vi "Teleop.vi"(10 "Match Info":T1={"Autonomous Elapsed Seconds"=0.0, "TeleOp Elapsed Seconds"=0.0, "Disabled Elapsed Seconds"=0.0, "Visited Autonomous"=FALSE, "Visited TeleOp"=FALSE, "Visited Disabled"=FALSE, "Autonomous Settings"={"Autonomous Style"=enum."Independent", "VI Refnum"=refnum}}, 11 "Call Context":T2) -> ()   [LabVIEW 2023]
doc: "This VI is called for each TeleOp packet received from the DS where the robot is not disabled. It is often used to read from the joysticks and update I/O or to update setpoints for timed control loops. It should complete and return within 20 milliseconds or it may miss DS packets."
uses:
  <vilib>/Rock Robotics/WPI/DriverStation/WPI_DriverStationDerivedRobotMode.ctl
  <vilib>/Rock Robotics/WPI/DriverStation/WPI_DriverStationMatch Info.ctl
  <vilib>/Rock Robotics/WPI/DriverStation/WPI_DriverStationAllianceInfo.ctl
  1688fe70-1696-4b7d-9b30-3e57ff5c803a.vi
  01ea3398-5322-4b29-8113-0a99e2c097c5.vi
  2d160a00-edc5-41ad-b49c-64d9a7043442.vi
  <vilib>/Rock Robotics/WPI/ThirdParty/JAS_Junk/TrajLib/ProfiledPIDController_NewPeriod.vi
  <vilib>/Rock Robotics/WPI/ThirdParty/JAS_Junk/TrajLib/ProfiledPIDController_SetIntegratorRange.vi
  <vilib>/Rock Robotics/WPI/ThirdParty/JAS_Junk/TrajLib/ProfiledPIDController_DisableContInput.vi
  <vilib>/Rock Robotics/WPI/ThirdParty/JAS_Junk/TrajLib/ProfiledPIDController_EnableContInput.vi
  <vilib>/Rock Robotics/WPI/ThirdParty/JAS_Junk/TrajLib/TrapProfConstraint_New.vi
  <vilib>/Rock Robotics/WPI/ThirdParty/PhotonVisionLib/SubVI/PhotonPipelineResult_Unpack.vi
  <vilib>/Rock Robotics/WPI/ThirdParty/PhotonVisionLib/SubVI/PhotonPipelineResult_SetTimeStampSecs.vi
  <vilib>/Rock Robotics/WPI/ThirdParty/PhotonVisionLib/SubVI/PhotonPipelineResult_GetLatency_Millis.vi
  <vilib>/Rock Robotics/WPI/ThirdParty/JAS_Junk/TrajLib/Util_GetTime.vi
  <vilib>/Rock Robotics/WPI/ThirdParty/PhotonVisionLib/SubVI/PhotonPipelineResult_GetTimeStampSecs.vi
  <vilib>/Rock Robotics/WPI/ThirdParty/JAS_Junk/TrajLib/MathUtil_AngleModulus.vi
  <vilib>/Rock Robotics/WPI/ThirdParty/JAS_Junk/TrajLib/Pose2d_New.vi
  <vilib>/Rock Robotics/WPI/ThirdParty/JAS_Junk/TrajLib/HolDrvCtrl_New.vi
  <vilib>/Rock Robotics/WPI/ThirdParty/JAS_Junk/TrajLib/HolDrvCtrl_PackPID.vi
  <vilib>/Rock Robotics/WPI/ThirdParty/JAS_Junk/TrajLib/HolDrvCtrl_SetTolerance.vi
  <vilib>/Rock Robotics/WPI/ThirdParty/JAS_Junk/TrajLib/HolDrvCtrl_SetEnabled.vi
  <vilib>/Rock Robotics/WPI/ThirdParty/JAS_Junk/TrajLib/HolDrvCtrl_AtReference.vi
  <vilib>/Rock Robotics/WPI/ThirdParty/JAS_Junk/TrajLib/HolDrvCtrl_Calculate.vi
  <vilib>/Rock Robotics/WPI/ThirdParty/JAS_Junk/TrajLib/Rotation2d_RotateBy.vi
  <vilib>/Rock Robotics/WPI/ThirdParty/JAS_Junk/TrajLib/SlewRateLimiter_New.vi
  <vilib>/Rock Robotics/WPI/ThirdParty/JAS_Junk/TrajLib/SlewRateLimiter_Reset.vi
  <vilib>/Rock Robotics/WPI/ThirdParty/JAS_Junk/TrajLib/SlewRateLimiter_Calculate.vi
  <vilib>/Rock Robotics/WPI/ThirdParty/JAS_Junk/TrajLib/SlewRateLimiter_SetRate.vi
  <vilib>/Rock Robotics/WPI/ThirdParty/JAS_Junk/TrajLib/Rotation2d_GetCos.vi
  <vilib>/Rock Robotics/WPI/ThirdParty/JAS_Junk/TrajLib/Rotation2d_GetSin.vi
  <vilib>/Rock Robotics/WPI/ThirdParty/JAS_Junk/TrajLib/ChassisSpeeds_New.vi
  <vilib>/Rock Robotics/WPI/ThirdParty/JAS_Junk/TrajLib/TrapProfState_New.vi
  <vilib>/Rock Robotics/WPI/ThirdParty/JAS_Junk/TrajLib/PIDController_NewPeriod.vi
  <vilib>/Rock Robotics/SystemInterfaces/NetworkCommunication/NetComm_UsageReport_report.vi
  <vilib>/Rock Robotics/WPI/ThirdParty/JAS_Junk/TrajLib/PIDController_SetIntegratorRange.vi
  <vilib>/Rock Robotics/WPI/ThirdParty/JAS_Junk/TrajLib/PIDController_DisableContinousInput.vi
  <vilib>/Rock Robotics/WPI/ThirdParty/JAS_Junk/TrajLib/PIDController_EnableContinousInput.vi
  <vilib>/Rock Robotics/WPI/ThirdParty/PhotonVisionLib/SubVI/Packet_decode_Flt64.vi
  <vilib>/Rock Robotics/WPI/ThirdParty/PhotonVisionLib/SubVI/Packet_decode_ByteI8.vi
  <vilib>/Rock Robotics/WPI/ThirdParty/PhotonVisionLib/SubVI/PhotonTrackedTarget_Unpack.vi
  <vilib>/Rock Robotics/WPI/ThirdParty/PhotonVisionLib/SubVI/PhotonMultiTargetPNPResult_unpack.vi
  <vilib>/Rock Robotics/WPI/ThirdParty/PhotonVisionLib/SubVI/PhotonPipelineResult_New.vi
  <vilib>/Rock Robotics/WPI/ThirdParty/JAS_Junk/TrajLib/VI/Util_GetTime_U32.vi
  <vilib>/Rock Robotics/WPI/ThirdParty/JAS_Junk/TrajLib/MathUtil_InputModulus.vi
  <vilib>/Rock Robotics/WPI/ThirdParty/JAS_Junk/TrajLib/Translation2d_Create.vi
  <vilib>/Rock Robotics/WPI/ThirdParty/JAS_Junk/TrajLib/PIDController_Reset.vi
  <vilib>/Rock Robotics/WPI/ThirdParty/JAS_Junk/TrajLib/Pose2d_getXYAngle.vi
  <vilib>/Rock Robotics/WPI/ThirdParty/JAS_Junk/TrajLib/Rotation2d_GetRadians.vi
  <vilib>/Rock Robotics/WPI/ThirdParty/JAS_Junk/TrajLib/Rotation2d_GetAngleCosSin.vi
  <vilib>/Rock Robotics/WPI/ThirdParty/JAS_Junk/TrajLib/Pose2d_RelativeTo.vi
  <vilib>/Rock Robotics/WPI/ThirdParty/JAS_Junk/TrajLib/Pose2d_getRotation.vi
  <vilib>/Rock Robotics/WPI/ThirdParty/JAS_Junk/TrajLib/Rotation2d_Minus.vi
  <vilib>/Rock Robotics/WPI/ThirdParty/JAS_Junk/TrajLib/ProfiledPIDController_Calculate_Meas_Goal.vi
  <vilib>/Rock Robotics/WPI/ThirdParty/JAS_Junk/TrajLib/PIDController_Calculate_SP_PV.vi
  <vilib>/Rock Robotics/WPI/ThirdParty/JAS_Junk/TrajLib/ProfiledPIDController_Reset_PosOnly.vi
  <vilib>/Rock Robotics/WPI/ThirdParty/JAS_Junk/TrajLib/Rotation2d_CreateXY.vi
  <vilib>/Rock Robotics/WPI/ThirdParty/PhotonVisionLib/SubVI/TargetCorner_New.vi
  <vilib>/Rock Robotics/WPI/ThirdParty/PhotonVisionLib/SubVI/Packet_decode_Int32.vi
  <vilib>/Rock Robotics/WPI/ThirdParty/PhotonVisionLib/SubVI/Packet_decode_Transform3d.vi
  <vilib>/Rock Robotics/WPI/ThirdParty/PhotonVisionLib/SubVI/PhotonPNPResult_unpackt.vi
  <vilib>/Rock Robotics/WPI/ThirdParty/PhotonVisionLib/SubVI/PhotonMultiTargetPNPResult_New.vi
  <vilib>/Rock Robotics/WPI/ThirdParty/PhotonVisionLib/SubVI/PhotonMultiTargetPNPResult_MAX_IDS.vi
  <vilib>/Rock Robotics/WPI/ThirdParty/PhotonVisionLib/SubVI/Packet_decode_Int16.vi
  <vilib>/Rock Robotics/WPI/ThirdParty/JAS_Junk/TrajLib/Transform2d_Create_PosePose.vi
  <vilib>/Rock Robotics/WPI/ThirdParty/JAS_Junk/TrajLib/Pose2d_New_TRRO.vi
  <vilib>/Rock Robotics/WPI/ThirdParty/JAS_Junk/TrajLib/Rotation2d_UnaryMinus.vi
  <vilib>/Rock Robotics/WPI/ThirdParty/JAS_Junk/TrajLib/ProfiledPIDController_SetGoal_PosOnly.vi
  <vilib>/Rock Robotics/WPI/ThirdParty/JAS_Junk/TrajLib/ProfiledPIDController_Calculate_Meas.vi
  <vilib>/Rock Robotics/WPI/ThirdParty/JAS_Junk/TrajLib/PIDController_SetSetpoint.vi
  <vilib>/Rock Robotics/WPI/ThirdParty/JAS_Junk/TrajLib/PIDController_Calculate_PV.vi
  <vilib>/Rock Robotics/WPI/ThirdParty/JAS_Junk/TrajLib/ProfiledPIDController_Reset.vi
  <vilib>/Rock Robotics/WPI/ThirdParty/JAS_Junk/TrajLib/Util_CalcDist.vi
  <vilib>/Rock Robotics/WPI/ThirdParty/JAS_Junk/TrajLib/VI/Transform3d_Create_Trans3dRot3d.vi
  <vilib>/Rock Robotics/WPI/ThirdParty/JAS_Junk/TrajLib/VI/Translation3d_Create.vi
  <vilib>/Rock Robotics/WPI/ThirdParty/JAS_Junk/TrajLib/VI/Rotation3d_Create_Quaternion.vi
  <vilib>/Rock Robotics/WPI/ThirdParty/JAS_Junk/TrajLib/VI/Quaternion_New.vi
  <vilib>/Rock Robotics/WPI/ThirdParty/PhotonVisionLib/SubVI/Packet_decode_Boolean.vi
  <vilib>/Rock Robotics/WPI/ThirdParty/PhotonVisionLib/SubVI/PhotonPNPResult_New_Empty.vi
  <vilib>/Rock Robotics/WPI/ThirdParty/PhotonVisionLib/SubVI/PhotonPNPResult_New.vi
  <vilib>/Rock Robotics/WPI/ThirdParty/JAS_Junk/TrajLib/Translation2d_RotateBy.vi
  <vilib>/Rock Robotics/WPI/ThirdParty/JAS_Junk/TrajLib/Translation2d_Minus.vi
  <vilib>/Rock Robotics/WPI/ThirdParty/JAS_Junk/TrajLib/ProfiledPIDController_SetGoal.vi
  <vilib>/Rock Robotics/WPI/ThirdParty/JAS_Junk/TrajLib/TrapProfile_New.vi
  <vilib>/Rock Robotics/WPI/ThirdParty/JAS_Junk/TrajLib/ProfiledPIDController_GetPeriod.vi
  <vilib>/Rock Robotics/WPI/ThirdParty/JAS_Junk/TrajLib/TrapProfile_Calculate.vi
  <vilib>/Rock Robotics/WPI/ThirdParty/JAS_Junk/TrajLib/ControllerUtil_GetModulusError.vi
  <vilib>/Rock Robotics/WPI/ThirdParty/JAS_Junk/TrajLib/VI/Quaternion_Normalize.vi
  <vilib>/Rock Robotics/WPI/ThirdParty/JAS_Junk/TrajLib/TrapProfile_ShouldFlipAcceleration.vi
  <vilib>/Rock Robotics/WPI/ThirdParty/JAS_Junk/TrajLib/TrapProfile_Direct.vi
  <vilib>/Rock Robotics/WPI/ThirdParty/JAS_Junk/TrajLib/PIDController_GetPeriod.vi
  <vilib>/Rock Robotics/WPI/ThirdParty/JAS_Junk/TrajLib/VI/Quaternion_New_Default.vi
  <vilib>/Rock Robotics/Network Tables/NT Read Boolean.vi
  <vilib>/Rock Robotics/Network Tables/NT Read Number.vi
  <vilib>/Rock Robotics/WPI/Utilities/WPI_GetSetVariantRefNum.vi
  <vilib>/Rock Robotics/Network Tables/NT Write Boolean Array.vi
  <vilib>/Rock Robotics/Network Tables/NT Write Numeric Array.vi
  <vilib>/Rock Robotics/Network Tables/NT Write String.vi
  <vilib>/Rock Robotics/Network Tables/NT Read String.vi
  <vilib>/Rock Robotics/Network Tables/NT Write Boolean.vi
  <vilib>/Rock Robotics/Network Tables/NT Write Number.vi
  <vilib>/Rock Robotics/WPI/ThirdParty/JAS_Junk/TrajLib/Globals/Util_LibraryGlobals.vi
  <vilib>/Rock Robotics/Network Tables/NT Read Raw.vi
  <vilib>/Rock Robotics/WPI/ThirdParty/JAS_Junk/TrajLib/VI/Util_GetTime_U64.vi
  Swerve_Drive_System/SWERVE_DRIVE_GLOBALS.vi
  <vilib>/addons/control/pid/pid.llb/PID Control Input Filter (DBL).vi
  <vilib>/Rock Robotics/WPI/ThirdParty/JAS_Junk/TrajLib/Trajectory_Library.lvlib
  55d04a09-3dfb-4cd7-90e5-cf451b4756f2.vi
  <vilib>/addons/control/pid/NI_PID_pid.lvlib
  <vilib>/Rock Robotics/WPI/ThirdParty/PhotonVisionLib/PhotonVisionLib.lvlib
panel:
  out "Sample Slider 0":dbl(slide) scale=0.0..5.0
  out "Sample Boolean 1":bool
  out "Sample Boolean 0":bool
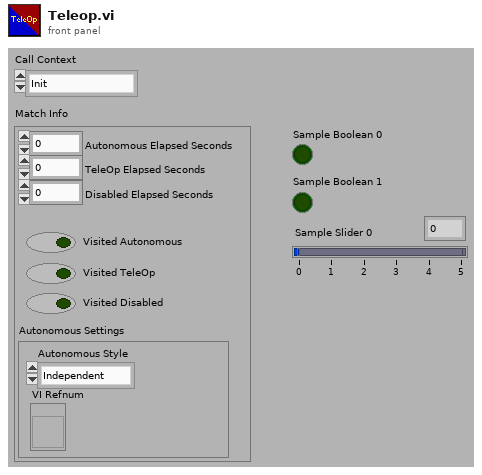
[diagram p1: front panel]
types:
  T1 = typedef "WPI_DriverStationMatch Info.ctl" = cluster{"Autonomous Elapsed Seconds":dbl, "TeleOp Elapsed Seconds":dbl, "Disabled Elapsed Seconds":dbl, "Visited Autonomous":bool, "Visited TeleOp":bool, "Visited Disabled":bool, "Autonomous Settings":cluster{"Autonomous Style":enum16{"Iterative", "Independent"}, "VI Refnum":refnum<vi>}}
  T2 = typedef "WPI_DriverStationDerivedRobotMode.ctl" = enum16{"Init", "Execute", "Stop"}
  T3 = typedef "WPI_JoystickDevRef.ctl" = cluster{"Device":T4}
  T4 = typedef "WPI_JoystickDeviceEnum.ctl" = enum16{"USB 0", "USB 1", "USB 2", "USB 3", "USB 4", "USB 5"}
  T5 = typedef "Trajectory_Library.lvlib/PID_TUNING.ctl" = cluster{"Kp":dbl, "Ki":dbl, "Kd":dbl, "MaximumIntegral":dbl, "MinimumIntegral":dbl, "IntegralZone":dbl}
  T6 = typedef "Trajectory_Library.lvlib/PROFILED_PID_CONTROLLER.ctl" = cluster{"Controller":T7, "Goal":T8, "Setpoint":T8, "Constraint":T9}
  T7 = typedef "Trajectory_Library.lvlib/PID_CONTROLLER.ctl" = cluster{"Kp":dbl, "Ki":dbl, "Kd":dbl, "Period":dbl, "Max_Integral":dbl, "Min_Integral":dbl, "Max_Input":dbl, "Min_Input":dbl, "Continuous":bool, "PositionError":dbl, "VelocityError":dbl, "PrevError":dbl, "Total_Integral":dbl, "PositionTolerance":dbl, "VelocityTolerance":dbl, "SetPoint":dbl, "Kf":dbl, "Prev_Deriv":dbl, "Prev_Deriv 2":dbl, "DerivativeFilter":bool, "Min_Output":dbl, "Max_Output":dbl, "Prev_F_P":dbl, "Prev_F_P_2":dbl, "AntiWindupActive":bool, "Measurement":dbl, "IntegralZone":dbl}
  T8 = typedef "Trajectory_Library.lvlib/TRAPEZOID_PROFILE_STATE.ctl" = cluster{"Position":dbl, "Velocity":dbl}
  T9 = typedef "Trajectory_Library.lvlib/TRAPEZOID_PROFILE_CONSTRAINT.ctl" = cluster{"MaxVelocity":dbl, "MaxAcceleration":dbl}
  T10 = typedef "Trajectory_Library.lvlib/HOLONOMIC_PACK_TUNING.ctl" = cluster{"X PID Tuning":T5, "Y PID Tuning":T5, "thetaProfiledPID_CTRL":T6}
  T11 = typedef "WPI_DriverStationAllianceInfo.ctl" = enum16{"Red", "Blue", "Invalid"}
  T12 = typedef "PhotonVisionLib.lvlib/PhotonPipelineResultType.ctl" = cluster{"TargetCount":i32, "Latency_MilliSec":dbl, "Targets":T13[], "TimeStampSec":dbl, "PhotonMultiTargetPNPResult":T19}
  T13 = typedef "PhotonVisionLib.lvlib/PhotonTrackedTargetType.ctl" = cluster{"Yaw":dbl, "Pitch":dbl, "Area":dbl, "Skew":dbl, "MinAreaRectCorners":T14[], "BestCameraToTarget":T15, "FiiducialId":i32, "AltCameraToTarget":T15, "PoseAmbiguity":dbl, "DetectedCorners":T14[]}
  T14 = typedef "PhotonVisionLib.lvlib/TargetCornerType.ctl" = cluster{"X":dbl, "Y":dbl}
  T15 = typedef "Trajectory_Library.lvlib/TRANSFORM3D.ctl" = cluster{"TRANSLATION3D":T16, "ROTATION3D":T17, "XF":bool}
  T16 = typedef "Trajectory_Library.lvlib/TRANSLATION3D.ctl" = cluster{"X":dbl, "Y":dbl, "Z":dbl}
  T17 = typedef "Trajectory_Library.lvlib/ROTATION3D.ctl" = cluster{"Q_quaternion":T18}
  T18 = typedef "Trajectory_Library.lvlib/QUATERNION.ctl" = cluster{"R":dbl, "V":dbl[]}
  T19 = typedef "PhotonVisionLib.lvlib/PhotonMultiTargetPNPResultType.ctl" = cluster{"PhotonPNPResult":T20, "FiducialIDsUsed":i16[]}
  T20 = typedef "PhotonVisionLib.lvlib/PhotonPNPResultType.ctl" = cluster{"IsPresent":bool, "bestReprojErr":dbl, "altReprojErr":dbl, "ambiguity":dbl, "Best":T15, "Alt":T15}
  T21 = typedef "Trajectory_Library.lvlib/SWERVE_DRIVE_POSE_EST2.ctl" = cluster{"M_Vision_K":T22, "m_nominal_dT":dbl, "m_PrevTime_Sec":dbl, "Pose_Buffer":T23, "Swerve_Drive_Kinematics":T24, "Swerve_Drive_Odom":T28, "M_Q":T22, "NumModules":i32}
  T22 = typedef "NI_Matrix.lvlib/RealMatrix.ctl" = dbl[][]
  T23 = typedef "Trajectory_Library.lvlib/TIME_INTERPOLATABLE_VARIANT.ctl" = cluster{"TimeStamps":dbl[], "DataArray":variant[], "Min_TimeStamp":dbl, "Max_TimeStamp":dbl, "ItemCount":i32, "MaxBufferTime":dbl}
  T24 = typedef "Trajectory_Library.lvlib/SWERVE_DRIVE_KINEMATICS.ctl" = cluster{"NumModules":i32, "InverseKinematics":T22, "ForwardKinematics":T22, "Modules":T25[], "PrevCoR":T25, "SavedModuleStates":T26[]}
  T25 = typedef "Trajectory_Library.lvlib/TRANSLATION2D.ctl" = cluster{"X":dbl, "Y":dbl}
  T26 = typedef "Trajectory_Library.lvlib/SWERVE_DRIVE_MODULE_STATE.ctl" = cluster{"Speed":dbl, "Angle":T27}
  T27 = typedef "Trajectory_Library.lvlib/ROTATION2D.ctl" = cluster{"VALUE":dbl, "COS":dbl, "SIN":dbl}
  T28 = typedef "Trajectory_Library.lvlib/SWERVE_DRIVE_ODOMETRY.ctl" = cluster{"POSE":T29, "GyroOffset":T27, "PreviousAngle":T27, "PrevModulePositions":T30[], "NumModules":i32}
  T29 = typedef "Trajectory_Library.lvlib/POSE2D.ctl" = cluster{"TRANSLATION":T25, "ROTATION":T27}
  T30 = typedef "Trajectory_Library.lvlib/SWERVE_DRIVE_MODULE_POSITION.ctl" = cluster{"Distance":dbl, "Angle":T27, "P":bool}
  T31 = typedef "Trajectory_Library.lvlib/CHASSIS_SPEEDS.ctl" = cluster{"vX":dbl, "vY":dbl, "vOmega":dbl}
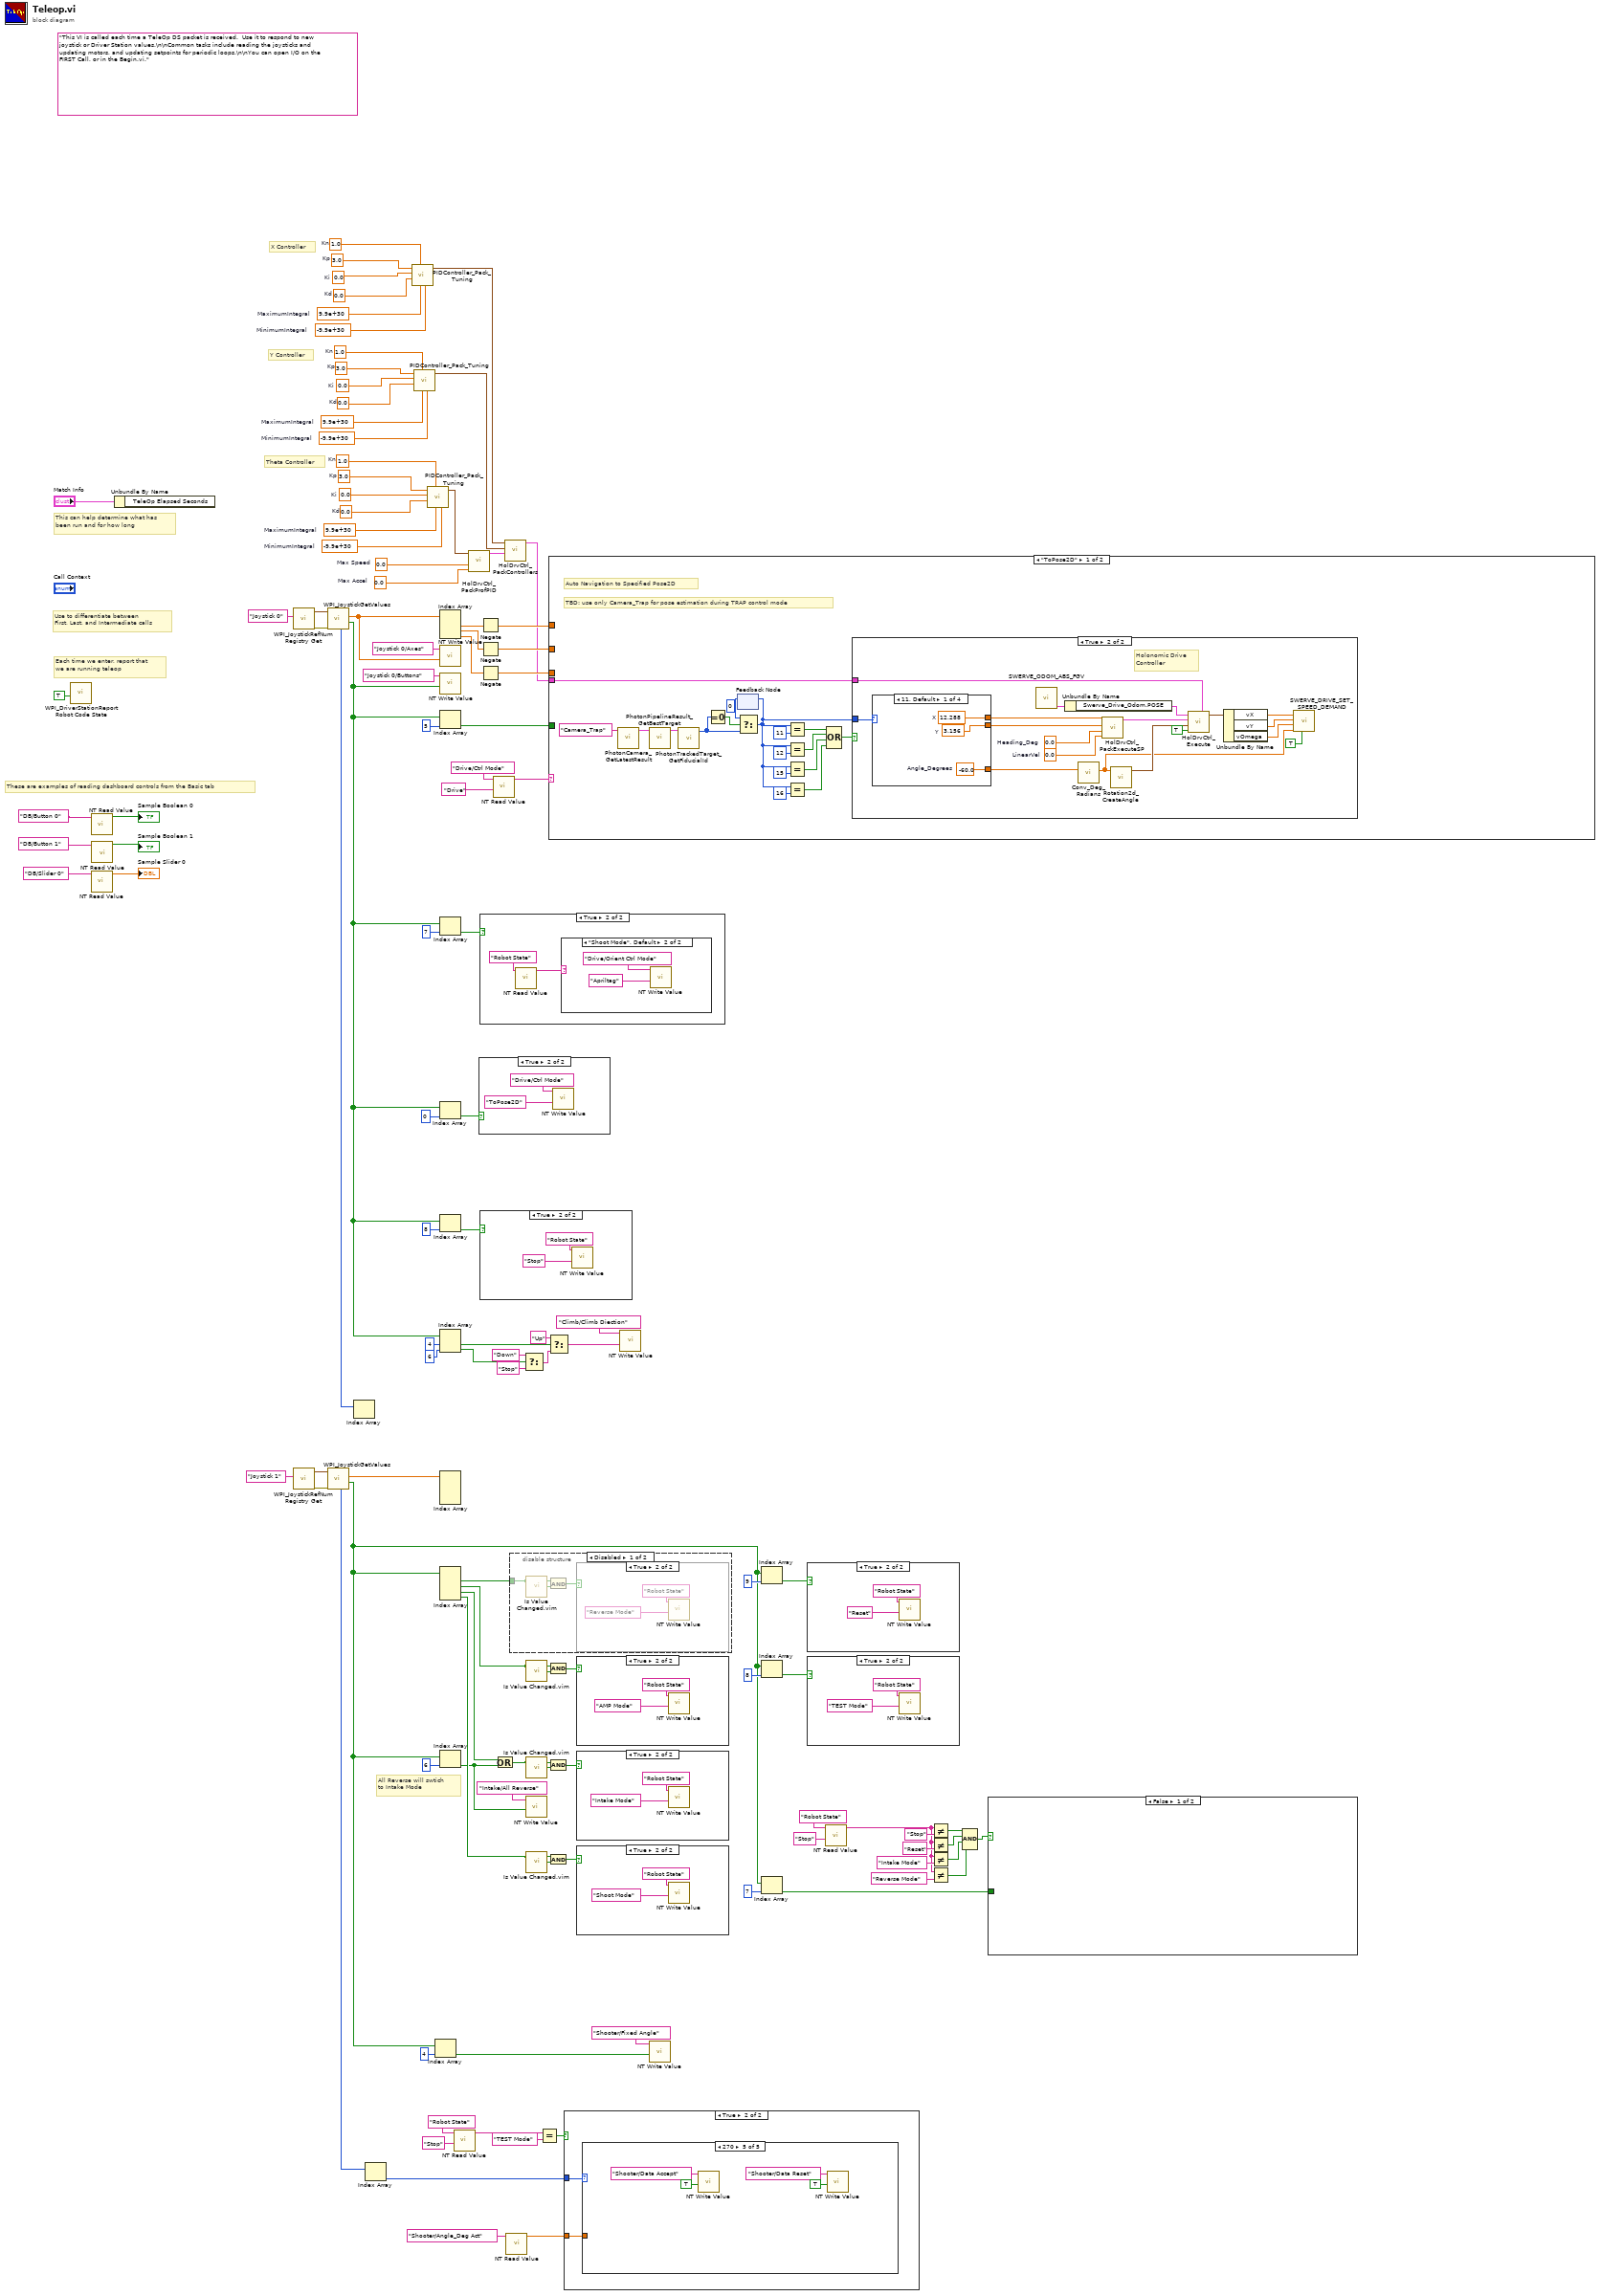
[diagram p0: block diagram]
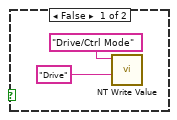
[diagram p4: hidden frame]
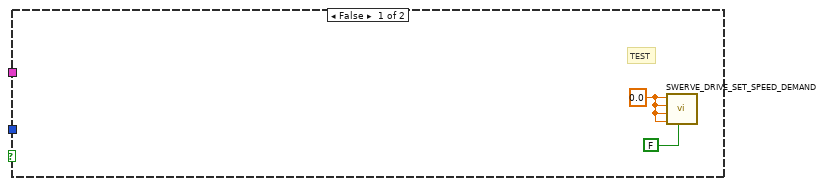
[diagram p5: hidden frame]
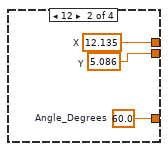
[diagram p6: hidden frame]
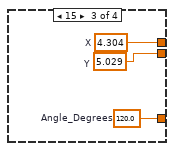
[diagram p7: hidden frame]
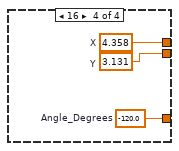
[diagram p8: hidden frame]
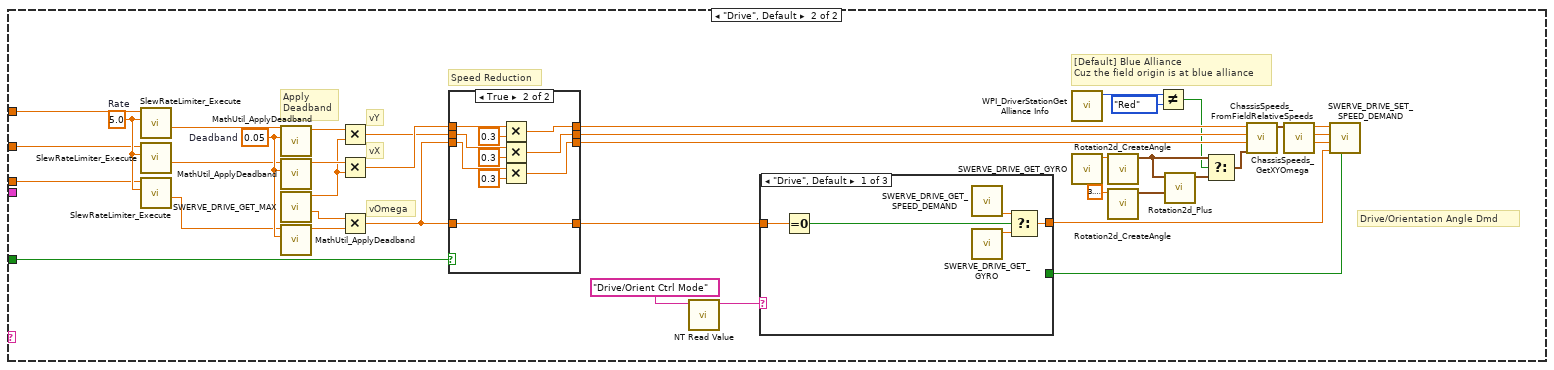
[diagram p9: hidden frame]
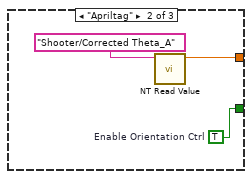
[diagram p11: hidden frame]
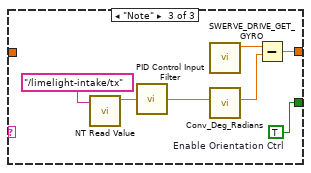
[diagram p12: hidden frame]
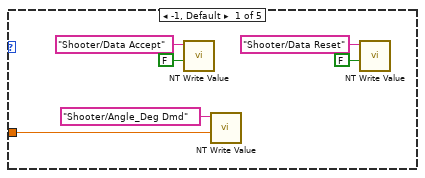
[diagram p14: hidden frame]
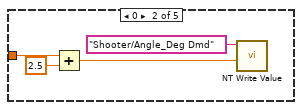
[diagram p15: hidden frame]
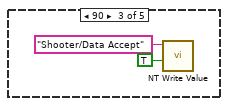
[diagram p16: hidden frame]
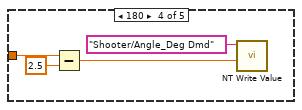
[diagram p17: hidden frame]
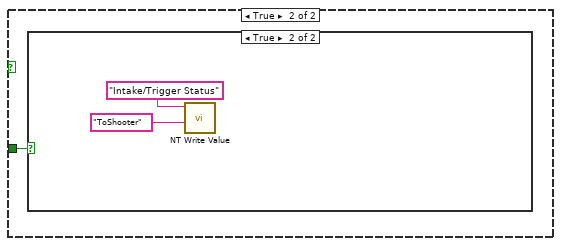
[diagram p18: hidden frame]
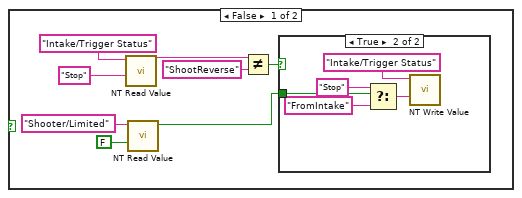
[diagram p19: hidden frame]
diagram:
  w10 = 1.0  # Kn
  w13 = 3.0  # Kp
  w22 = 0.0  # Ki
  w23 = 0.0  # Kd
  w24 = 9.9e+30  # MaximumIntegral
  w25 = -9.9e+30  # MinimumIntegral
  w8 = 1.0  # Kn
  w11 = 3.0  # Kp
  w14 = 0.0  # Ki
  w15 = 0.0  # Kd
  w16 = 9.9e+30  # MaximumIntegral
  w17 = -9.9e+30  # MinimumIntegral
  w9 = 1.0  # Kn
  w12 = 3.0  # Kp
  w18 = 0.0  # Ki
  w19 = 0.0  # Kd
  w20 = 9.9e+30  # MaximumIntegral
  w21 = -9.9e+30  # MinimumIntegral
  w7 = 0.0  # Max Accel
  w6 = 0.0  # Max Speed
  (unwired) "This VI is called each time a TeleOp DS packet is received.  Use it to respond to new joystick or Driver Station values.\n\nCommon tasks include reading the joysticks and updating motors, and updating setpoints for periodic loops.\n\nYou can open I/O on the FIRST Call, or in the Begin.vi."
  # "Theta Controller"
  # "Y Controller"
  # "X Controller"
  # "All Reverse will swtich \nto Intake Mode"
  # "These are examples of reading dashboard controls from the Basic tab"
  # "Each time we enter, report that\nwe are running teleop"
  # "Use to differentiate between\nFirst, Last, and Intermediate calls"
  # "This can help determine what has\nbeen run and for how long"
  n1 = call <vilib>:"WPI_DriverStationReport Robot Code State.vi"("TeleOp"=TRUE ("Autonomous")) -> ()  [unwired: 10 in, 1 out]
  n2 = call-poly <vilib>:"NT Read Value.vi"("name"="DB/Button 0" ("refnum name")) -> ("value"=→"Sample Boolean 0":bool)  [unwired: 8 in, 2 out]
  n3 = call-poly <vilib>:"NT Read Value.vi"("name"="DB/Slider 0" ("refnum name")) -> ("value"=→"Sample Slider 0":dbl)  [unwired: 8 in, 2 out]
  n4 = call-poly <vilib>:"NT Read Value.vi"("name"="DB/Button 1" ("refnum name")) -> ("value"=→"Sample Boolean 1":bool)  [unwired: 8 in, 2 out]
  n5 = Unbundle By Name("Match Info") -> ()  [unwired: 1 out]
  n6 = call <vilib>:"WPI_JoystickRefNum Registry Get.vi"("refnum name"="Joystick 0") -> ("error out"=w97:errorcluster, "JoystickDevRef"=w108:T3)  [unwired: 1 in, 8 out]
  n7 = call <vilib>:"WPI_JoystickRefNum Registry Get.vi"("refnum name"="Joystick 1") -> ("error out"=w93:errorcluster, "JoystickDevRef"=w95:T3)  [unwired: 1 in, 8 out]
  n8 = call <vilib>:"WPI_JoystickGetValues.vi"("error in (no error)"=w97, "JoystickDevRef"=w108) -> ("Buttons"=w33:bool[], "Axes"=w104:dbl[], "POVs"=w105:i16[])  [unwired: 5 in, 2 out]
  n9 = call <vilib>:"WPI_JoystickGetValues.vi"("error in (no error)"=w93, "JoystickDevRef"=w95) -> ("Buttons"=w55:bool[], "Axes"=w94:dbl[], "POVs"=w72:i16[])  [unwired: 5 in, 2 out]
  n10 = Index Array(array=w105) -> ()  [unwired: 1 in, 1 out]
  n11 = Index Array(array=w72) -> (element=w73:i16)  [unwired: 1 in]
  n12 = call <vilib>:"PIDController_Pack_Tuning.vi"("MinimumIntegral"=w17, "MaximumIntegral"=w16, "Kn"=w8, "Kd"=w15, "Ki"=w14, "Kp"=w11) -> ("PID Tuning"=w26:T5)  [unwired: 5 in]
  n13 = call <vilib>:"PIDController_Pack_Tuning.vi"("MinimumIntegral"=w21, "MaximumIntegral"=w20, "Kn"=w9, "Kd"=w19, "Ki"=w18, "Kp"=w12) -> ("PID Tuning"=w28:T5)  [unwired: 5 in]
  n14 = call <vilib>:"PIDController_Pack_Tuning.vi"("MinimumIntegral"=w25, "MaximumIntegral"=w24, "Kn"=w10, "Kd"=w23, "Ki"=w22, "Kp"=w13) -> ("PID Tuning"=w5:T5)  [unwired: 5 in]
  n15 = Index Array(array=w55, index=4) -> (element=w42:bool)
  n16 = Index Array(array=w33, index=0) -> (element=w32:bool)
  n17 = Index Array(array=w104) -> (element #1=w102:dbl, element #2=w103:dbl, element #3=w101:dbl)  [unwired: 3 in]
  n18 = call-poly <vilib>:"NT Write Value.vi"("value"=w104, "name"="Joystick 0/Axes" ("Name")) -> ()  [unwired: 9 in, 1 out]
  n19 = call-poly <vilib>:"NT Write Value.vi"("value"=w33, "name"="Joystick 0/Buttons" ("Name")) -> ()  [unwired: 9 in, 1 out]
  n20 = Index Array(array=w33, index=5) -> (element=w56:bool)
  n21 = Index Array(array=w33, index=7) -> (element=w65:bool)
  n22 = Index Array(array=w33, index=8) -> (element=w76:bool)
  n23 = Index Array(array=w33, index #1=4 ("index"), index #2=6 ("index")) -> (element #1=w45:bool, element #2=w48:bool)
  n24 = Index Array(array=w94) -> ()  [unwired: 4 in, 4 out]
  n25 = Index Array(array=w55) -> (element #1=w92:bool, element #2=w90:bool, element #3=w70:bool, element #4=w87:bool)  [unwired: 4 in]
  n26 = Index Array(array=w55, index=6) -> (element=w69:bool)
  n27 = call-poly <vilib>:"NT Read Value.vi"("default value"="Stop", "name"="Robot State") -> ("value"=w37:string)  [unwired: 7 in, 2 out]
  n28 = call <vilib>:"HolDrvCtrl_PackProfPID.vi"("Max Accel"=w7, "Max Speed"=w6, "Theta PID Tuning"=w5) -> ("Theta PID CONTROLLER"=w27:T6)  [unwired: 8 in]
  n29 = case shown="True" w32 {
    frame False {
      n30 = call-poly <vilib>:"NT Write Value.vi"("value"="Drive" ("default value"), "name"="Drive/Ctrl Mode") -> ()  [unwired: 9 in, 1 out]
    }
    frame True {
      n31 = call-poly <vilib>:"NT Write Value.vi"("value"="ToPose2D" ("default value"), "name"="Drive/Ctrl Mode") -> ()  [unwired: 9 in, 1 out]
    }
  }
  n32 = Negate(x=w102) -> (-x=w100:dbl)
  n33 = Negate(x=w103) -> (-x=w99:dbl)
  n34 = Negate(x=w101) -> (-x=w98:dbl)
  n35 = case shown="True" w65 {
    frame False {
      n36 = call-poly <vilib>:"NT Write Value.vi"("value"="Drive" ("default value"), "name"="Drive/Orient Ctrl Mode") -> ()  [unwired: 9 in, 1 out]
    }
    frame True {
      n37 = call-poly <vilib>:"NT Read Value.vi"("name"="Robot State") -> ("value"=w124:string)  [unwired: 8 in, 2 out]
      n38 = case shown="\"Shoot Mode\", Default" w124 {
        frame "Intake Mode" {
          n39 = call-poly <vilib>:"NT Write Value.vi"("value"="Note" ("default value"), "name"="Drive/Orient Ctrl Mode") -> ()  [unwired: 9 in, 1 out]
        }
        frame "Shoot Mode", Default {
          n40 = call-poly <vilib>:"NT Write Value.vi"("value"="Apriltag" ("default value"), "name"="Drive/Orient Ctrl Mode") -> ()  [unwired: 9 in, 1 out]
        }
      }
    }
  }
  n41 = case shown="True" w76 {
    frame False {
    }
    frame True {
      n42 = call-poly <vilib>:"NT Write Value.vi"("value"="Stop" ("default value"), "name"="Robot State") -> ()  [unwired: 9 in, 1 out]
    }
  }
  n43 = call-poly <vilib>:"NT Read Value.vi"("default value"="Drive", "name"="Drive/Ctrl Mode") -> ("value"=w29:string)  [unwired: 7 in, 2 out]
  n44 = Or(x=w70, y=w69) -> (x .or. y?=w71:bool)
  n45 = call <vilib>:"HolDrvCtrl_PackControllers.vi"("thetaProfiledPID_CTRL"=w27, "Y PID Tuning"=w28, "X PID Tuning"=w26) -> ("HOLONOMIC_CTRL_PACK_TUNING"=w4:T10)  [unwired: 8 in]
  n46 = call-poly <vilib>:"NT Read Value.vi"("name"="Shooter/Angle_Deg Act") -> ("value"=w40:dbl)  [unwired: 8 in, 2 out]
  n47 = disable-structure shown="Disabled" {
    disable-tunnel: w92 -> [w133 _]
    frame Disabled {
      n48 = call "Is Value Changed.vim"("value"=w133) -> ("changed or first call?"=w134:bool)
      n49 = And(x=w133, y=w134) -> (x .and. y?=w132:bool)
      n50 = case shown="True" w132 {
        frame False {
        }
        frame True {
          n51 = call-poly <vilib>:"NT Write Value.vi"("value"="Reverse Mode" ("default value"), "name"="Robot State") -> ()  [unwired: 9 in, 1 out]
        }
      }
    }
    frame Enabled {
    }
  }
  n52 = Select(t="Down", s=w48, f="Stop" ("default value")) -> (s? t:f=w51:string)
  n53 = call-poly <vilib>:"NT Write Value.vi"("value"=w69, "name"="Intake/All Reverse") -> ()  [unwired: 9 in, 1 out]
  n54 = call "Is Value Changed.vim"("value"=w90) -> ("changed or first call?"=w91:bool)
  n55 = call "Is Value Changed.vim"("value"=w71) -> ("changed or first call?"=w89:bool)
  n56 = call "Is Value Changed.vim"("value"=w87) -> ("changed or first call?"=w88:bool)
  n57 = Equal?(x=w37, y="TEST Mode") -> (x = y?=w35:bool)
  n58 = And(x=w90, y=w91) -> (x .and. y?=w84:bool)
  n59 = And(x=w71, y=w89) -> (x .and. y?=w85:bool)
  n60 = And(x=w87, y=w88) -> (x .and. y?=w86:bool)
  n61 = case shown="\"ToPose2D\"" w29 {
    tunnel: w100 -> [_ w217]
    tunnel: w99 -> [_ w215]
    tunnel: w98 -> [_ w213]
    tunnel: w56 -> [_ w196]
    tunnel: w4 -> [w154 _]
    frame "ToPose2D" {
      # "TBD: use only Camera_Trap for pose estimation during TRAP control mode"
      # "Auto Navigation to Specified Pose2D"
      n62 = call <vilib>:"PhotonCamera_GetLatestResult.vi"("CameraName"="Camera_Trap") -> ("PipelineResult"=w153:T12)  [unwired: 7 in, 3 out]
      n63 = call <vilib>:"PhotonPipelineResult_GetBestTarget.vi"("PhotonPipelineResult"=w153) -> ("PhotonTrackedTarget"=w152:T13)  [unwired: 9 in, 1 out]
      n64 = call <vilib>:"PhotonTrackedTarget_GetFiducialId.vi"("TrackedTarget"=w152) -> ("Fiducial Id"=w140:i32)  [unwired: 10 in]
      n65 = Equal To 0?(x=w140) -> (x = 0?=w141:bool)
      n66 = feedback #1(0 ("Fiducial Id")) -> (w139:i32)
      n67 = Select(t=w139, s=w141, f=w140) -> (s? t:f=w137:i32)
      n68 = feedback-in #1(w137) -> ()
      n69 = Equal?(x=w137, y=11) -> (x = y?=w143:bool)
      n70 = Equal?(x=w137, y=12) -> (x = y?=w146:bool)
      n71 = Equal?(x=w137, y=15) -> (x = y?=w145:bool)
      n72 = Equal?(x=w137, y=16) -> (x = y?=w144:bool)
      n73 = Compound Arithmetic op=OR(w143, w146, w145, w144) -> (w142:bool)
      n74 = case shown="True" w142 {
        tunnel: w154 -> [_ w163]
        tunnel: w137 -> [_ w160]
        frame False {
          w156 = 0.0 ("Drv X Vel Dmd")
          # "TEST"
          n75 = call "SWERVE_DRIVE_SET_SPEED_DEMAND.vi"("Enable Orientation Ctrl? (False)"=FALSE, "Drv Rotation Orentation Dmd"=w156, "Drv Angular Vel Dmd"=w156, "Drv Y Vel Dmd"=w156, "Drv X Vel Dmd"=w156) -> ()  [unwired: 7 in]
        }
        frame True {
          w164 = 0.0  # Heading_Deg
          w170 = 0.0  # LinearVel
          # "Holonomic Drive\nController"
          n76 = case shown="11, Default" w160 {
            tunnel: [w177 w180 w183 w186] -> w162
            tunnel: [w176 w179 w182 w185] -> w161
            tunnel: [w175 w178 w181 w184] -> w159
            frame 11, Default {
              w175 = -60.0  # Angle_Degrees
              w176 = 3.156  # Y
              w177 = 12.288  # X
            }
            frame 12 {
              w178 = 60.0  # Angle_Degrees
              w179 = 5.086  # Y
              w180 = 12.135  # X
            }
            frame 15 {
              w181 = 120.0  # Angle_Degrees
              w182 = 5.029  # Y
              w183 = 4.304  # X
            }
            frame 16 {
              w184 = -120.0  # Angle_Degrees
              w185 = 3.131  # Y
              w186 = 4.358  # X
            }
          }
          n77 = call "SWERVE_ODOM_ABS_FGV.vi"() -> ("out SWERVE_DRIVE_POSE_EST2"=w173:T21)  [unwired: 10 in, 1 out]
          n78 = Unbundle By Name(w173) -> ("Swerve_Drive_Odom.POSE"=w172:T29)
          n79 = call <vilib>:"Conv_Deg_Radians.vi"("Degress"=w159) -> ("Radians"=w158:dbl)  [unwired: 10 in]
          n80 = call <vilib>:"HolDrvCtrl_PackExecuteSP.vi"("LinearVel"=w170, "Heading_Deg"=w164, "Y"=w161, "X"=w162) -> ("HolExecuteSP"=w174:cluster{"DesiredPose":T29, "LinearVel":dbl})  [unwired: 7 in]
          n81 = call <vilib>:"Rotation2d_CreateAngle.vi"("Angle"=w158) -> ("ROTATION"=w171:T27)  [unwired: 10 in]
          n82 = call <vilib>:"HolDrvCtrl_Execute.vi"("HOLONOMIC_CTRL_PACK_TUNING"=w163, "Enable"=TRUE, "angleRef"=w171, "HolExecuteSP"=w174, "currentPose"=w172) -> ("calcChassisSpeed"=w168:T31)  [unwired: 4 in, 2 out]
          n83 = Unbundle By Name(w168) -> ("vX"=w167:dbl, "vY"=w166:dbl, "vOmega"=w165:dbl)
          n84 = call "SWERVE_DRIVE_SET_SPEED_DEMAND.vi"("Enable Orientation Ctrl? (False)"=TRUE, "Drv Rotation Orentation Dmd"=w158, "Drv Angular Vel Dmd"=w165, "Drv Y Vel Dmd"=w166, "Drv X Vel Dmd"=w167) -> ()  [unwired: 7 in]
        }
      }
    }
    frame "Drive", Default {
      w218 = 5.0  # Rate
      w224 = 0.05  # Deadband
      # "Speed Reduction"
      # "[Default] Blue Alliance\nCuz the field origin is at blue alliance"
      # "Drive/Orientation Angle Dmd"
      # "vOmega"
      # "vX"
      # "vY"
      # "Apply\nDeadband"
      n85 = call <vilib>:"SlewRateLimiter_Execute.vi"("PositiveRate"=w218, "Input"=w217) -> ("Output"=w216:dbl)  [unwired: 8 in, 1 out]
      n86 = call <vilib>:"SlewRateLimiter_Execute.vi"("PositiveRate"=w218, "Input"=w215) -> ("Output"=w214:dbl)  [unwired: 8 in, 1 out]
      n87 = call <vilib>:"SlewRateLimiter_Execute.vi"("PositiveRate"=w218, "Input"=w213) -> ("Output"=w212:dbl)  [unwired: 8 in, 1 out]
      n88 = call <vilib>:"MathUtil_ApplyDeadband.vi"("Deadband"=w224, "Value"=w216) -> ("Result"=w223:dbl)  [unwired: 9 in]
      n89 = call <vilib>:"MathUtil_ApplyDeadband.vi"("Deadband"=w224, "Value"=w214) -> ("Result"=w222:dbl)  [unwired: 9 in]
      n90 = call "SWERVE_DRIVE_GET_MAX.vi"() -> ("Max Rotational Vel (Rad/Sec)"=w220:dbl, "Max Wheel Vel (Meter/Sec)"=w221:dbl)  [unwired: 10 in]
      n91 = call <vilib>:"MathUtil_ApplyDeadband.vi"("Deadband"=w224, "Value"=w212) -> ("Result"=w219:dbl)  [unwired: 9 in]
      n92 = Multiply(x=w223, y=w221) -> (x*y=w194:dbl)
      n93 = Multiply(x=w222, y=w221) -> (x*y=w195:dbl)
      n94 = Multiply(x=w220, y=w219) -> (x*y=w193:dbl)
      n95 = case shown="True" w196 {
        tunnel: w195 -> [w227 w237]
        tunnel: w194 -> [w226 w236]
        tunnel: w193 -> [w225 w234]
        tunnel: w193 -> [w228 w238]
        tunnel: [w228 w238] -> w192
        tunnel: [w227 w229] -> w191
        tunnel: [w226 w230] -> w190
        tunnel: [w225 w231] -> w189
        frame False {
        }
        frame True {
          n96 = Multiply(x=w237, y=0.3) -> (x*y=w229:dbl)
          n97 = Multiply(x=w236, y=0.3) -> (x*y=w230:dbl)
          n98 = Multiply(x=w234, y=0.3) -> (x*y=w231:dbl)
        }
      }
      n99 = call-poly <vilib>:"NT Read Value.vi"("name"="Drive/Orient Ctrl Mode") -> ("value"=w204:string)  [unwired: 8 in, 2 out]
      n100 = case shown="\"Drive\", Default" w204 {
        tunnel: w192 -> [w243 _ _]
        tunnel: [w242 w245 w253] -> w206
        tunnel: [_ w244 w247] -> w187
        frame "Drive", Default {
          n101 = Equal To 0?(x=w243) -> (x = 0?=w240:bool)
          n102 = call "SWERVE_DRIVE_GET_SPEED_DEMAND.vi"() -> ("Drv Rotation Orentation Dmd"=w239:dbl)  [unwired: 7 in, 4 out]
          n103 = call "SWERVE_DRIVE_GET_GYRO.vi"() -> ("Gyro Heading Radians"=w241:dbl)  [unwired: 11 in]
          n104 = Select(t=w239, s=w240, f=w241) -> (s? t:f=w242:dbl)
        }
        frame "Apriltag" {
          w244 = TRUE  # Enable Orientation Ctrl
          n105 = call-poly <vilib>:"NT Read Value.vi"("name"="Shooter/Corrected Theta_A") -> ("value"=w245:dbl)  [unwired: 8 in, 2 out]
        }
        frame "Note" {
          w247 = TRUE  # Enable Orientation Ctrl
          n106 = call-poly <vilib>:"NT Read Value.vi"("name"="/limelight-intake/tx") -> ("value"=w249:dbl)  [unwired: 8 in, 2 out]
          n107 = call-poly <vilib>:"PID Control Input Filter.vi"("input"=w249) -> ("output"=w248:dbl)  [unwired: 4 in]
          n108 = call "SWERVE_DRIVE_GET_GYRO.vi"() -> ("Gyro Heading Radians"=w252:dbl)  [unwired: 11 in]
          n109 = call <vilib>:"Conv_Deg_Radians.vi"("Degress"=w248) -> ("Radians"=w251:dbl)  [unwired: 10 in]
          n110 = Subtract(x=w252, y=w251) -> (x-y=w253:dbl)
        }
      }
      n111 = call <vilib>:"WPI_DriverStationGet Alliance Info.vi"() -> ("Alliance"=w203:T11)  [unwired: 6 in, 5 out]
      n112 = call "SWERVE_DRIVE_GET_GYRO.vi"() -> ("Gyro Heading Radians"=w210:dbl)  [unwired: 11 in]
      n113 = call <vilib>:"Rotation2d_CreateAngle.vi"("Angle"=w210) -> ("ROTATION"=w199:T27)  [unwired: 10 in]
      n114 = call <vilib>:"Rotation2d_CreateAngle.vi"("Angle"=3.141592653589793) -> ("ROTATION"=w200:T27)  [unwired: 10 in]
      n115 = Not Equal?(x=w203, y=WPI_DriverStationAllianceInfo."Red") -> (x != y?=w188:bool)
      n116 = call <vilib>:"Rotation2d_Plus.vi"("other ROTATION"=w200, "in ROTATION"=w199) -> ("out ROTATION"=w197:T27)  [unwired: 9 in]
      n117 = Select(t=w199, s=w188, f=w197) -> (s? t:f=w198:T27)
      n118 = call <vilib>:"ChassisSpeeds_FromFieldRelativeSpeeds.vi"("RobotAngle"=w198, "Omega"=w189, "vY"=w190, "vX"=w191) -> ("CHASSIS"=w211:T31)  [unwired: 7 in]
      n119 = call <vilib>:"ChassisSpeeds_GetXYOmega.vi"("CHASSIS"=w211) -> ("vAngular"=w207:dbl, "vY"=w208:dbl, "vX"=w209:dbl)  [unwired: 8 in]
      n120 = call "SWERVE_DRIVE_SET_SPEED_DEMAND.vi"("Enable Orientation Ctrl? (False)"=w187, "Drv Rotation Orentation Dmd"=w206, "Drv Angular Vel Dmd"=w207, "Drv Y Vel Dmd"=w208, "Drv X Vel Dmd"=w209) -> ()  [unwired: 7 in]
    }
  }
  n121 = Select(t="Up", s=w45, f=w51) -> (s? t:f=w49:string)
  n122 = case shown="True" w35 {
    tunnel: w73 -> [_ w255]
    tunnel: w40 -> [_ w254]
    frame False {
    }
    frame True {
      n123 = case shown="270" w255 {
        tunnel: w254 -> [w260 w262 _ w268 _]
        frame -1, Default {
          n124 = call-poly <vilib>:"NT Write Value.vi"("value"=FALSE, "name"="Shooter/Data Accept") -> ()  [unwired: 9 in, 1 out]
          n125 = call-poly <vilib>:"NT Write Value.vi"("value"=w260, "name"="Shooter/Angle_Deg Dmd") -> ()  [unwired: 9 in, 1 out]
          n126 = call-poly <vilib>:"NT Write Value.vi"("value"=FALSE, "name"="Shooter/Data Reset") -> ()  [unwired: 9 in, 1 out]
        }
        frame 0 {
          n127 = Add(x=w262, y=2.5) -> (x+y=w263:dbl)
          n128 = call-poly <vilib>:"NT Write Value.vi"("value"=w263, "name"="Shooter/Angle_Deg Dmd") -> ()  [unwired: 9 in, 1 out]
        }
        frame 90 {
          n129 = call-poly <vilib>:"NT Write Value.vi"("value"=TRUE, "name"="Shooter/Data Accept") -> ()  [unwired: 9 in, 1 out]
        }
        frame 180 {
          n130 = Subtract(x=w268, y=2.5) -> (x-y=w269:dbl)
          n131 = call-poly <vilib>:"NT Write Value.vi"("value"=w269, "name"="Shooter/Angle_Deg Dmd") -> ()  [unwired: 9 in, 1 out]
        }
        frame 270 {
          n132 = call-poly <vilib>:"NT Write Value.vi"("value"=TRUE, "name"="Shooter/Data Accept") -> ()  [unwired: 9 in, 1 out]
          n133 = call-poly <vilib>:"NT Write Value.vi"("value"=TRUE, "name"="Shooter/Data Reset") -> ()  [unwired: 9 in, 1 out]
        }
      }
    }
  }
  n134 = case shown="True" w84 {
    frame False {
    }
    frame True {
      n135 = call-poly <vilib>:"NT Write Value.vi"("value"="AMP Mode" ("default value"), "name"="Robot State") -> ()  [unwired: 9 in, 1 out]
    }
  }
  n136 = case shown="True" w85 {
    frame False {
    }
    frame True {
      n137 = call-poly <vilib>:"NT Write Value.vi"("value"="Intake Mode" ("default value"), "name"="Robot State") -> ()  [unwired: 9 in, 1 out]
    }
  }
  n138 = case shown="True" w86 {
    frame False {
    }
    frame True {
      n139 = call-poly <vilib>:"NT Write Value.vi"("value"="Shoot Mode" ("default value"), "name"="Robot State") -> ()  [unwired: 9 in, 1 out]
    }
  }
  n140 = call-poly <vilib>:"NT Write Value.vi"("value"=w49, "name"="Climb/Climb Diection") -> ()  [unwired: 9 in, 1 out]
  n141 = call-poly <vilib>:"NT Write Value.vi"("value"=w42, "name"="Shooter/Fixed Angle") -> ()  [unwired: 9 in, 1 out]
  n142 = Index Array(array=w55, index=9) -> (element=w82:bool)
  n143 = Index Array(array=w55, index=8) -> (element=w68:bool)
  n144 = Index Array(array=w55, index=7) -> (element=w59:bool)
  n145 = case shown="True" w82 {
    frame False {
    }
    frame True {
      n146 = call-poly <vilib>:"NT Write Value.vi"("value"="Reset" ("default value"), "name"="Robot State") -> ()  [unwired: 9 in, 1 out]
    }
  }
  n147 = case shown="True" w68 {
    frame False {
    }
    frame True {
      n148 = call-poly <vilib>:"NT Write Value.vi"("value"="TEST Mode" ("default value"), "name"="Robot State") -> ()  [unwired: 9 in, 1 out]
    }
  }
  n149 = call-poly <vilib>:"NT Read Value.vi"("default value"="Stop", "name"="Robot State") -> ("value"=w2:string)  [unwired: 7 in, 2 out]
  n150 = Not Equal?(x=w2, y="Stop") -> (x != y?=w62:bool)
  n151 = Not Equal?(x=w2, y="Reset") -> (x != y?=w61:bool)
  n152 = Not Equal?(x=w2, y="Intake Mode") -> (x != y?=w60:bool)
  n153 = Not Equal?(x=w2, y="Reverse Mode") -> (x != y?=w1:bool)
  n154 = Compound Arithmetic op=AND(w62, w61, w60, w1) -> (w58:bool)
  n155 = case shown="False" w58 {
    tunnel: w59 -> [_ w286]
    frame False {
    }
    frame True {
      n156 = case shown="True" w286 {
        frame False {
          n157 = call-poly <vilib>:"NT Read Value.vi"("default value"="Stop", "name"="Intake/Trigger Status") -> ("value"=w293:string)  [unwired: 7 in, 2 out]
          n158 = call-poly <vilib>:"NT Read Value.vi"("default value"=FALSE ("value"), "name"="Shooter/Limited") -> ("value"=w287:bool)  [unwired: 7 in, 2 out]
          n159 = Not Equal?(x=w293, y="ShootReverse" ("default value")) -> (x != y?=w290:bool)
          n160 = case shown="True" w290 {
            tunnel: w287 -> [_ w296]
            frame False {
            }
            frame True {
              n161 = Select(t="Stop" ("default value"), s=w296, f="FromIntake") -> (s? t:f=w295:string)
              n162 = call-poly <vilib>:"NT Write Value.vi"("value"=w295, "name"="Intake/Trigger Status") -> ()  [unwired: 9 in, 1 out]
            }
          }
        }
        frame True {
          n163 = call-poly <vilib>:"NT Write Value.vi"("value"="ToShooter" ("default value"), "name"="Intake/Trigger Status") -> ()  [unwired: 9 in, 1 out]
        }
      }
    }
  }
